vi "Lorentzian-Fitter v2.vi"() -> ()   [LabVIEW 2014]
doc: "Intended use:\n-Displays collected data\n-Attempts a fit to background; separates signal from background\n-Allows user to select a subarray of data with cursors\n-Fits the signal from this subarray to a specified function (in this case, a Lorentzian) and outputs the fit parameters"
uses:
  <vilib>/Utility/file.llb/Read From Spreadsheet File (DBL).vi
  <vilib>/gmath/NumericalOptimization/Nonlinear Curve Fit LM bound.vi
  <vilib>/gmath/NI_Gmath.lvlib
panel:
  out "best fit params":dbl[](array[numeric])
  out "initial params":dbl[](array[numeric])
  out "Subset and Fit":T1(graph)
  out "Data and BG":cluster{"all rows":dbl[], "all rows":dbl[]}[](graph)
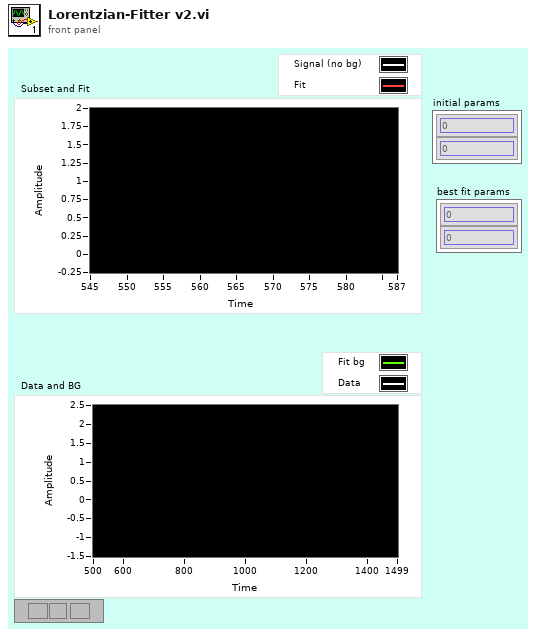
[diagram p1: front panel]
types:
  T1 = cluster{"X subset":dbl[], "best nonlinear fit":dbl[]}[]
  T2 = cluster{"parameter minimum":dbl[], "parameter maximum":dbl[]}
  T3 = typedef "eventvkey.ctl" = enum16{"ASCII", "Enter", "Return", "Shift", "Ctrl", "Alt", "Cmd", "Opt", "Caps", "NumLock", "Clear", "Break", "Up", "Down", "Left", "Right", "Insert", "Delete", "Home", "End", "PageUp", "PageDown", "Escape", "Help", "Pause", "ScrollLock", "F1", "F2", "F3", "F4", "F5", "F6", "F7", "F8", "F9", "F10", "F11", "F12", "F13", "F14", "F15", "F16", "F17", "F18", "F19", "F20", "F21", "F22", "F23", "F24", "Play", "VolumeUp", "VolumeDown", "Mute", "Two Byte Char"}
  T4 = cluster{"X subset":dbl[], "best nonlinear fit":dbl[]}
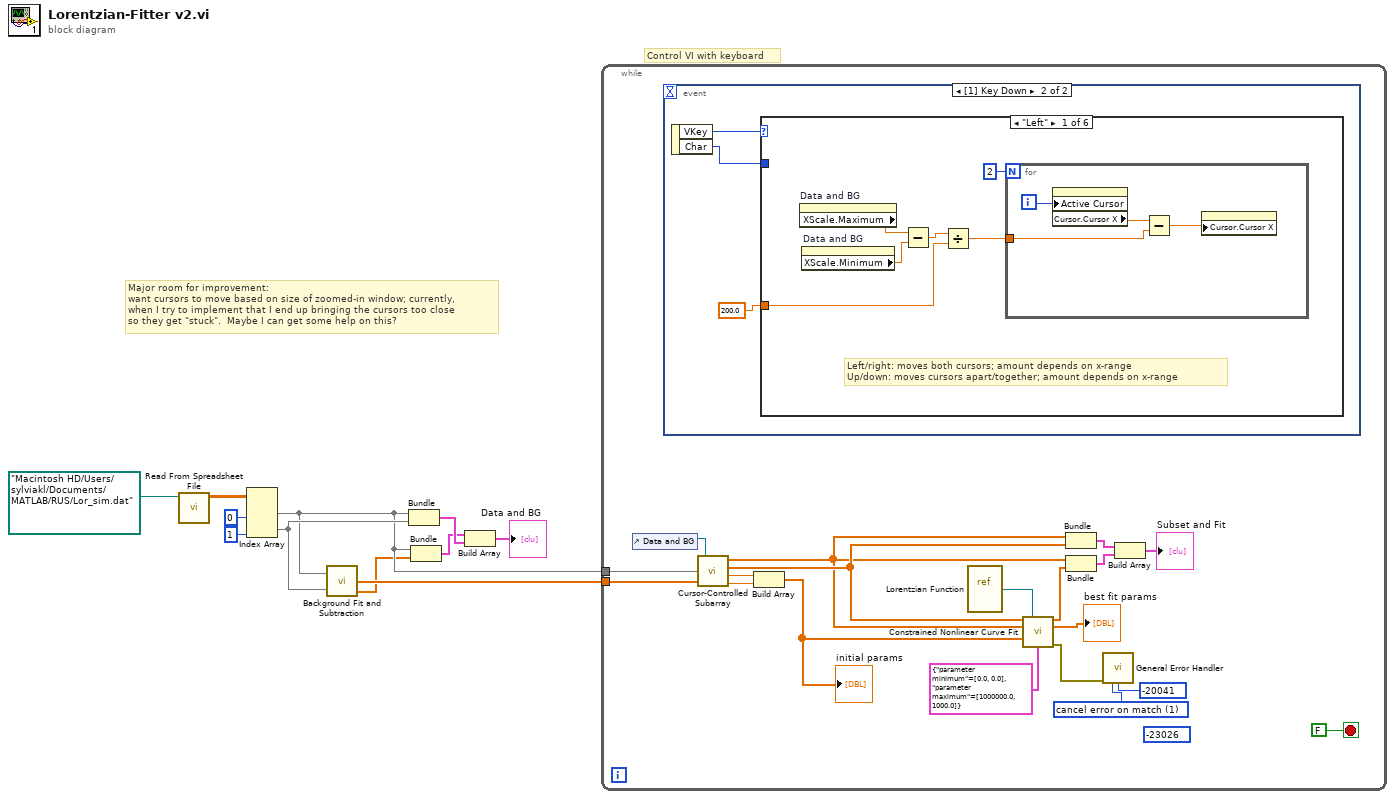
[diagram p0: block diagram]
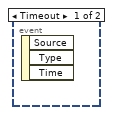
[diagram p2: hidden frame]
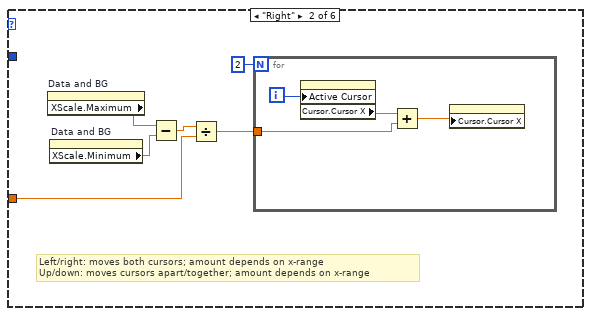
[diagram p3: hidden frame]
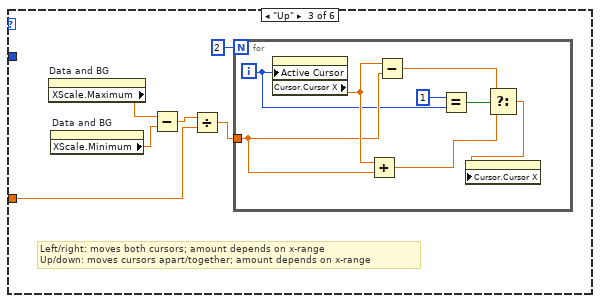
[diagram p4: hidden frame]
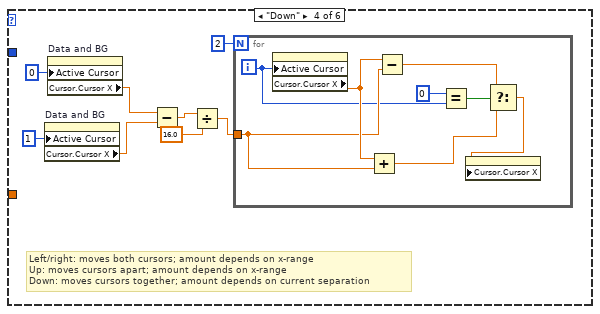
[diagram p5: hidden frame]
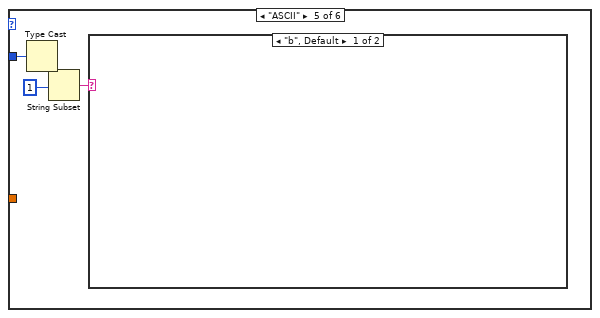
[diagram p6: hidden frame]
diagram:
  # "Major room for improvement:\nwant cursors to move based on size of zoomed-in window; currently,\nwhen I try to implement that I end up bringing the cursors too close\nso they get \"stuck\".  Maybe I can get some help on this?"
  # "Control VI with keyboard"
  n1 = call-poly <vilib>:"Read From Spreadsheet File.vi"("file path (dialog if empty)"=path "/Macintosh HD/Users/sylviakl/Documents/MATLAB/RUS/Lor_sim.dat") -> ("all rows"=w8:dbl[][])  [unwired: 6 in, 4 out]
  n2 = Index Array(array=w8, index (col) #1=0 ("disabled index (col)"), index (col) #2=1 ("index (col)")) -> (element #1=w6:dbl[], element #2=w7:dbl[])  [unwired: 2 in]
  n3 = call "Background Fit and Subtraction.vi"("X"=w6, "Y"=w7) -> ("signal"=w4:dbl[], "background"=w3:dbl[])  [unwired: 1 out]
  n4 = Bundle("all rows"=w6, "all rows"=w7) -> (w2:cluster{"all rows":dbl[], "all rows":dbl[]})  [unwired: 1 in]
  n5 = Bundle("all rows"=w6, "background"=w3) -> (w1:cluster{"all rows":dbl[], "background":dbl[]})  [unwired: 1 in]
  n6 = Build Array(w1, w2) -> (→"Data and BG":cluster{"all rows":dbl[], "all rows":dbl[]}[])
  n7 = while {
    tunnel: w6 -> [w20]
    tunnel: w4 -> [w19]
    stop <- FALSE stop-if-true
    (unwired) -23026 ("[exception code]")
    w24 = 1 items=["no exception", "cancel error on match", "set error on match"] ("[exception action] (none:0)")
    n8 = control-ref of="Data and BG"() -> (w17:refnum<vi>)
    n9 = event shown="[1] Key Down" {
      selector: _ -> [_ _]
      dyn-events: _ -> [_ _]
      timeout: _ -> [_ _]
      event Timeout {
        n10 = event-data() -> ()  [unwired: 1 in, 3 out]
      }
      event Key Down {
        n11 = event-data() -> ("VKey"=w33:T3, "Char"=w32:i16)  [unwired: 1 in]
        n12 = case shown="\"Left\"" w33 {
          tunnel: w32 -> [_ _ _ _ w87 _]
          tunnel: 200.0 ("y") -> [w34 w44 w54 _ _ _]
          frame "Left" {
            # "Left/right: moves both cursors; amount depends on x-range\nUp/down: moves cursors apart/together; amount depends on x-range"
            n13 = property on="Data and BG" class="XYGraph (strict)"() -> ("XScale.Maximum"=w37:dbl)  [unwired: 2 in, 2 out]
            n14 = property on="Data and BG" class="XYGraph (strict)"() -> ("XScale.Minimum"=w36:dbl)  [unwired: 2 in, 2 out]
            n15 = Subtract(x=w37, y=w36) -> (x-y=w38:dbl)
            n16 = Divide(x=w38, y=w34) -> (x/y=w35:dbl)
            n17 = for {
              N: 2 -> [_]
              tunnel: w35 -> [w40]
              i -> [w41]
              n18 = property on="Data and BG" class="XYGraph (strict)"("Active Cursor"=w41) -> ("Cursor.Cursor X"=w42:dbl)  [unwired: 2 in, 2 out]
              n19 = Subtract(x=w42, y=w40) -> (x-y=w43:dbl)
              n20 = property on="Data and BG" class="XYGraph (strict)"("Cursor.Cursor X"=w43) -> ()  [unwired: 2 in, 2 out]
            }
          }
          frame "Right" {
            # "Left/right: moves both cursors; amount depends on x-range\nUp/down: moves cursors apart/together; amount depends on x-range"
            n21 = property on="Data and BG" class="XYGraph (strict)"() -> ("XScale.Maximum"=w47:dbl)  [unwired: 2 in, 2 out]
            n22 = property on="Data and BG" class="XYGraph (strict)"() -> ("XScale.Minimum"=w46:dbl)  [unwired: 2 in, 2 out]
            n23 = Subtract(x=w47, y=w46) -> (x-y=w48:dbl)
            n24 = Divide(x=w48, y=w44) -> (x/y=w45:dbl)
            n25 = for {
              N: 2 -> [_]
              tunnel: w45 -> [w50]
              i -> [w51]
              n26 = property on="Data and BG" class="XYGraph (strict)"("Active Cursor"=w51) -> ("Cursor.Cursor X"=w52:dbl)  [unwired: 2 in, 2 out]
              n27 = Add(x=w52, y=w50) -> (x+y=w53:dbl)
              n28 = property on="Data and BG" class="XYGraph (strict)"("Cursor.Cursor X"=w53) -> ()  [unwired: 2 in, 2 out]
            }
          }
          frame "Up" {
            # "Left/right: moves both cursors; amount depends on x-range\nUp/down: moves cursors apart/together; amount depends on x-range"
            n29 = property on="Data and BG" class="XYGraph (strict)"() -> ("XScale.Maximum"=w57:dbl)  [unwired: 2 in, 2 out]
            n30 = property on="Data and BG" class="XYGraph (strict)"() -> ("XScale.Minimum"=w56:dbl)  [unwired: 2 in, 2 out]
            n31 = Subtract(x=w57, y=w56) -> (x-y=w58:dbl)
            n32 = Divide(x=w58, y=w54) -> (x/y=w55:dbl)
            n33 = for {
              N: 2 -> [_]
              tunnel: w55 -> [w66]
              i -> [w61]
              n34 = property on="Data and BG" class="XYGraph (strict)"("Active Cursor"=w61) -> ("Cursor.Cursor X"=w67:dbl)  [unwired: 2 in, 2 out]
              n35 = Add(x=w67, y=w66) -> (x+y=w64:dbl)
              n36 = Subtract(x=w67, y=w66) -> (x-y=w65:dbl)
              n37 = Equal?(x=1, y=w61) -> (x = y?=w62:bool)
              n38 = Select(t=w65, s=w62, f=w64) -> (s? t:f=w63:dbl)
              n39 = property on="Data and BG" class="XYGraph (strict)"("Cursor.Cursor X"=w63) -> ()  [unwired: 2 in, 2 out]
            }
          }
          frame "Down" {
            # "Left/right: moves both cursors; amount depends on x-range\nUp: moves cursors apart; amount depends on x-range\nDown: moves cursors together; amount depends on current separation"
            n40 = property on="Data and BG" class="XYGraph (strict)"("Active Cursor"=u32 1) -> ("Cursor.Cursor X"=w71:dbl)  [unwired: 2 in, 2 out]
            n41 = property on="Data and BG" class="XYGraph (strict)"("Active Cursor"=u32 0) -> ("Cursor.Cursor X"=w70:dbl)  [unwired: 2 in, 2 out]
            n42 = Subtract(x=w70, y=w71) -> (x-y=w74:dbl)
            n43 = Divide(x=w74, y=16.0) -> (x/y=w73:dbl)
            n44 = for {
              N: 2 -> [_]
              tunnel: w73 -> [w82]
              i -> [w77]
              n45 = property on="Data and BG" class="XYGraph (strict)"("Active Cursor"=w77) -> ("Cursor.Cursor X"=w83:dbl)  [unwired: 2 in, 2 out]
              n46 = Add(x=w83, y=w82) -> (x+y=w80:dbl)
              n47 = Subtract(x=w83, y=w82) -> (x-y=w81:dbl)
              n48 = Equal?(x=0, y=w77) -> (x = y?=w78:bool)
              n49 = Select(t=w81, s=w78, f=w80) -> (s? t:f=w79:dbl)
              n50 = property on="Data and BG" class="XYGraph (strict)"("Cursor.Cursor X"=w79) -> ()  [unwired: 2 in, 2 out]
            }
          }
          frame "ASCII" {
            n51 = Type Cast(x=w87) -> (*(type *) &x=w86:string)  [unwired: 1 in]
            n52 = String Subset(string=w86, offset (0)=1) -> (substring=w84:string)  [unwired: 1 in]
            n53 = case shown="\"b\", Default" w84 {
              frame "b", Default {
              }
              frame "a" {
              }
            }
          }
          frame Default {
          }
        }
      }
    }
    n54 = call "Cursor-Controlled Subarray.vi"("cursor graph"=w17, "X"=w20, "Y"=w19) -> ("X subset"=w15:dbl[], "Y subset"=w16:dbl[], "cursor avg"=w13:dbl, "cursor diff"=w14:dbl)
    n55 = Build Array(w13, w14) -> (w26:dbl[])
    "initial params" <- w26
    n56 = vi-ref "Lorentzian Function.vi"() -> (w12:refnum<vi>)
    n57 = call-poly <vilib>:"Constrained Nonlinear Curve Fit.vi"("Y"=w16, "f(x,a)"=w12, "X"=w15, "initial parameters"=w26, "parameter bounds"=T2 {"parameter minimum"=[0.0, 0.0], "parameter maximum"=[1000000.0, 1000.0]}) -> ("best nonlinear fit"=w23:dbl[], "best fit parameters"=→"best fit params":dbl[], "error out"=w21:errorcluster)  [unwired: 5 in, 3 out]
    n58 = Bundle("X subset"=w15, "Y subset"=w16) -> (w28:cluster{"X subset":dbl[], " Y subset":dbl[]})  [unwired: 1 in]
    n59 = Bundle("X subset"=w15, "best nonlinear fit"=w23) -> (w27:T4)  [unwired: 1 in]
    n60 = call <vilib>:"General Error Handler.vi"("error in (no error)"=w21, "[exception action] (none:0)"=w24, "[exception code]"=-20041) -> ()  [unwired: 8 in, 5 out]
    n61 = Build Array(w28, w27) -> (→"Subset and Fit":T1)
  }
